vi "SQL读取.vi"(8 "error in (no error)":errorcluster caption="错误输入（无错误）", 10 "ADODB._Connection In":refnum<k7>, 11 "电脑一新返工1":string) -> (0 "error out":errorcluster caption="错误输出", 1 "computer3":string, 2 "computer2":string, 3 "computer1":string, 4 "传递信息显示":string, 5 "ADODB._Connection Out":refnum<k7>)   [LabVIEW 2017]
uses:
  <vilib>/Utility/file.llb/Write Delimited Spreadsheet (string).vi
panel:
  out "工单号":string
  out "元素 3":string
  out "元素 2":string
  out "元素":string
  out "连接的字符串":string
  out "Data":string[][](array[string])
  out "子数组":string[](array[string])
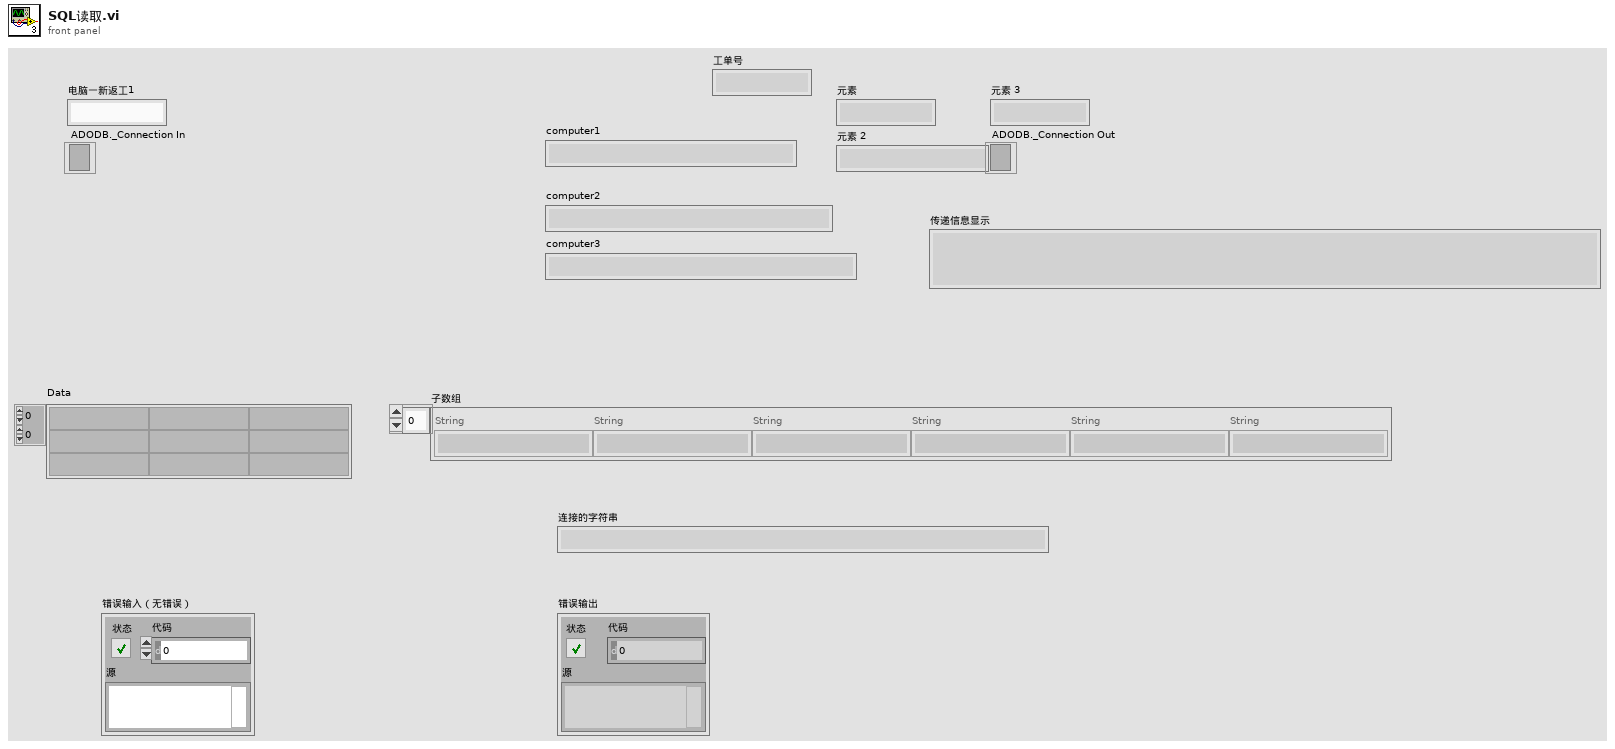
[diagram p1: front panel]
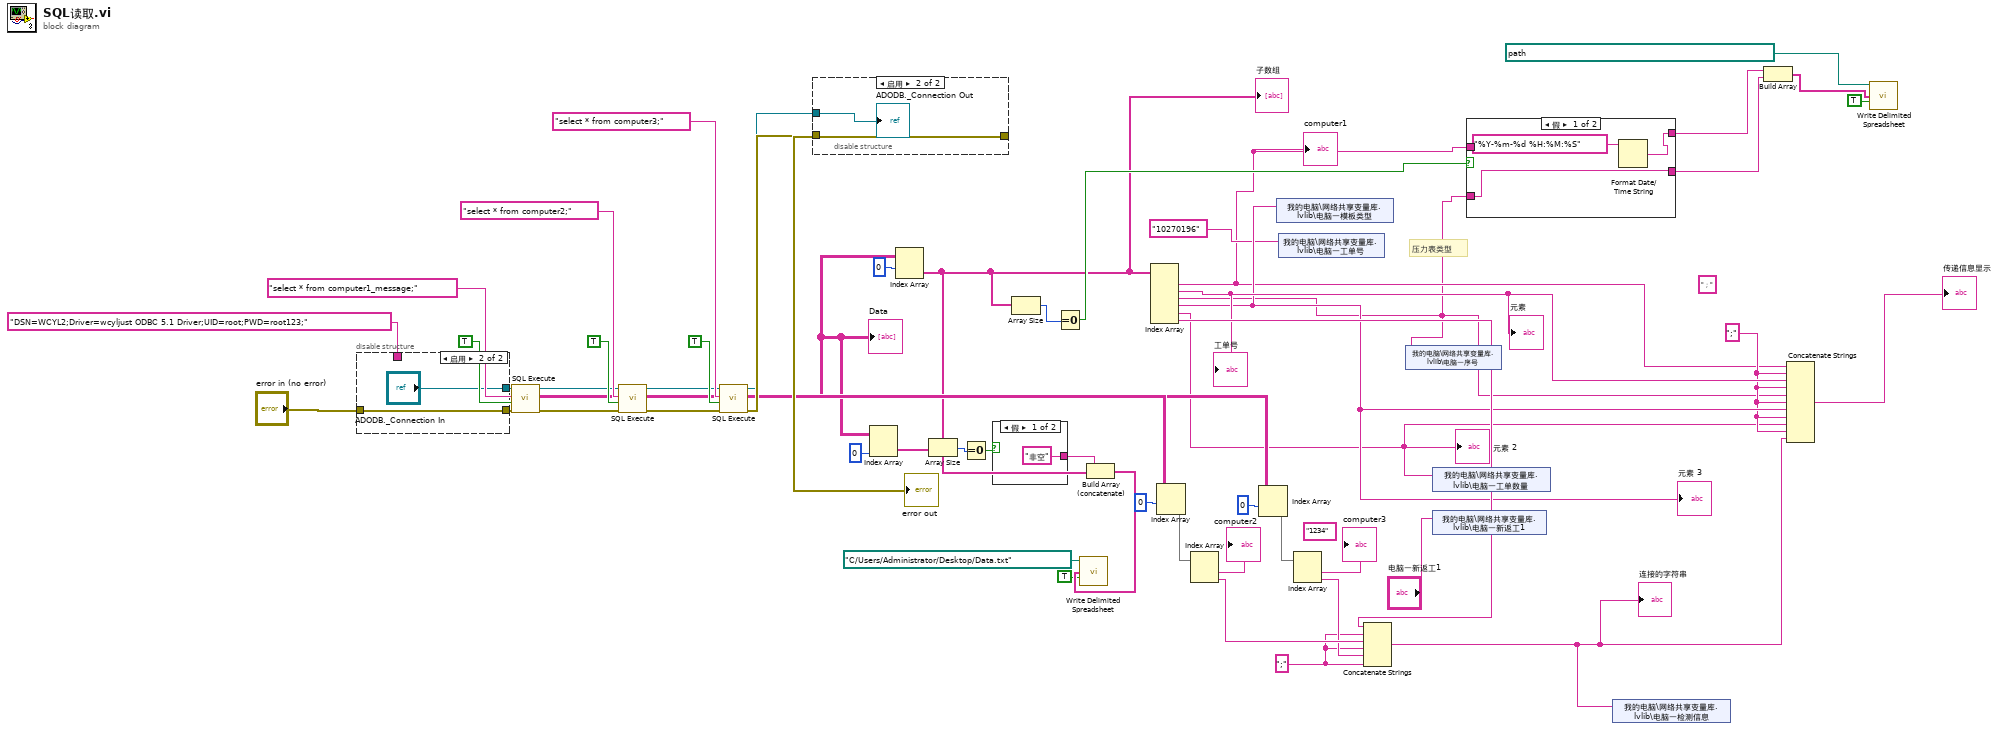
[diagram p0: block diagram]
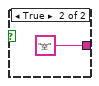
[diagram p2: hidden frame]
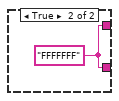
[diagram p3: hidden frame]
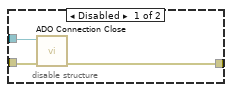
[diagram p4: hidden frame]
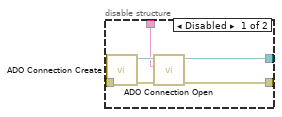
[diagram p5: hidden frame]
diagram:
  (unwired) "1234" ("电脑一返工")
  w22 = ";" ("字符串")
  (unwired) "；" ("字符串")
  w32 = ";" ("字符串")
  # "压力表类型"
  n1 = disable-structure shown="启用" {
    disable-tunnel: "DSN=WCYL2;Driver=wcyljust ODBC 5.1 Driver;UID=root;PWD=root123;" ("ConnectionString") -> [w61 _]
    disable-tunnel: [w60 "ADODB._Connection In"] -> w53
    disable-tunnel: [w59 w65] -> w52
    disable-tunnel: "error in (no error)" -> [w58 w65]
    frame Disabled {
      n2 = call <userlib>:"ADO Connection Create.vi"("error in (no error)"=w58) -> ("error out"=w62:errorcluster, "ADODB._Connection Out"=w63:refnum<k7>)  [unwired: 9 in]
      n3 = call <userlib>:"ADO Connection Open.vi"("error in (no error)"=w62, "ConnectionString"=w61, "ADODB._Connection In"=w63) -> ("error out"=w59:errorcluster, "ADODB._Connection Out"=w60:refnum<k7>)  [unwired: 7 in]
    }
    frame Enabled {
    }
  }
  n4 = call <userlib>:"SQL Execute.vi"("error in (no error)"=w52, "Return Data (T)"=TRUE, "Command Text"="select * from computer1_message;", "ADODB._Connection In"=w53) -> ("error out"=w45:errorcluster, "Data"=w9:string[][], "ADODB._Connection Out"=w42:refnum<k7>)  [unwired: 4 in, 1 out]
  "Data" <- w9
  n5 = call <userlib>:"SQL Execute.vi"("error in (no error)"=w45, "Return Data (T)"=TRUE, "Command Text"="select * from computer2;", "ADODB._Connection In"=w42) -> ("error out"=w44:errorcluster, "Data"=w39:string[][], "ADODB._Connection Out"=w41:refnum<k7>)  [unwired: 4 in, 1 out]
  n6 = call <userlib>:"SQL Execute.vi"("error in (no error)"=w44, "Return Data (T)"=TRUE, "Command Text"="select * from computer3;", "ADODB._Connection In"=w41) -> ("error out"=w43:errorcluster, "Data"=w38:string[][], "ADODB._Connection Out"=w40:refnum<k7>)  [unwired: 4 in, 1 out]
  n7 = disable-structure shown="启用" {
    disable-tunnel: [w68 w70] -> w50
    disable-tunnel: w43 -> [w67 w70]
    disable-tunnel: w40 -> [w66 w69]
    frame Disabled {
      n8 = call <userlib>:"ADO Connection Close.vi"("error in (no error)"=w67, "ADODB._Connection In"=w66) -> ("error out"=w68:errorcluster)  [unwired: 8 in, 1 out]
    }
    frame Enabled {
      "ADODB._Connection Out" <- w69
    }
  }
  "error out" <- w50
  n9 = Index Array(array=w9, index (col)=0 ("禁用的索引 (列)")) -> (element=w7:string[])  [unwired: 1 in]
  n10 = Index Array(array=w9, index (row)=0 ("索引 (行)")) -> (element=w3:string[])  [unwired: 1 in]
  "子数组" <- w3
  n11 = Array Size(array=w7) -> (size(s)=w6:i32)
  n12 = Equal To 0?(x=w6) -> (x = 0?=w5:bool)
  n13 = case shown="假" w5 {
    tunnel: ["非空" "空"] -> w4
    frame False {
    }
    frame True {
    }
  }
  n14 = Array Size(array=w3) -> (size(s)=w16:i32)
  n15 = Equal To 0?(x=w16) -> (x = 0?=w15:bool)
  n16 = Build Array (concatenate)(w4, w3) -> (w2:string[])
  n17 = call-poly <vilib>:"Write Delimited Spreadsheet.vi"("file path (dialog if empty)"=path "C:/Users/Administrator/Desktop/Data.txt", "1D data"=w2, "append to file? (new file:F)"=TRUE) -> ()  [unwired: 11 in, 2 out]
  n18 = Index Array(array=w3) -> (element #1=w14:string, element #2=w36:string, element #3=w12:string, element #4=w33:string, element #5=w31:string, element #6=w37:string)  [unwired: 6 in]
  "computer1" <- w14
  "元素" <- w36
  "元素 2" <- w31
  "元素 3" <- w33
  "工单号" <- w36
  n19 = Index Array(array=w39, index (row)=0 ("索引 (行)")) -> (element=w28:string[])  [unwired: 1 in]
  n20 = Index Array(array=w28) -> (element #1=→"computer2":string, element #2=w26:string)  [unwired: 2 in]
  n21 = Index Array(array=w38, index (row)=0 ("索引 (行)")) -> (element=w27:string[])  [unwired: 1 in]
  n22 = shared-variable "我的电脑\\网络共享变量库.lvlib\\电脑一模板类型"(w33) -> ()  [unwired: 1 in, 1 out]
  n23 = shared-variable "我的电脑\\网络共享变量库.lvlib\\电脑一工单号"("10270196" ("电脑一工单号")) -> ()  [unwired: 1 in, 1 out]
  n24 = Index Array(array=w27) -> (element #1=→"computer3":string, element #2=w25:string)  [unwired: 2 in]
  n25 = Concatenate Strings(w37, w22, w26, w22, w25, w22) -> (w35:string)
  "连接的字符串" <- w35
  n26 = shared-variable "我的电脑\\网络共享变量库.lvlib\\电脑一序号"(w12) -> ()  [unwired: 1 in, 1 out]
  n27 = shared-variable "我的电脑\\网络共享变量库.lvlib\\电脑一工单数量"(w31) -> ()  [unwired: 1 in, 1 out]
  n28 = shared-variable "我的电脑\\网络共享变量库.lvlib\\电脑一新返工1"("电脑一新返工1") -> ()  [unwired: 1 in, 1 out]
  n29 = case shown="假" w15 {
    tunnel: [w73 w76] -> w13
    tunnel: w14 -> [_ _]
    tunnel: [w75 w76] -> w11
    tunnel: w12 -> [w75 _]
    frame False {
      n30 = Format Date/Time String(time format string (%c)="%Y-%m-%d %H:%M:%S" ("时间格式字符串(%c)")) -> (date/time string=w73:string)  [unwired: 2 in]
    }
    frame True {
      w76 = "FFFFFFF" ("String")
    }
  }
  n31 = shared-variable "我的电脑\\网络共享变量库.lvlib\\电脑一检测信息"(w35) -> ()  [unwired: 1 in, 1 out]
  n32 = Build Array(w13, w11) -> (w17:string[])
  n33 = Concatenate Strings(w14, w32, w36, w32, w12, w32, w33, w32, w31, w32, w35) -> (→"传递信息显示":string)
  n34 = call-poly <vilib>:"Write Delimited Spreadsheet.vi"("file path (dialog if empty)"=path "C:/Users/Administrator/Desktop/传递条码信息.txt", "1D data"=w17, "append to file? (new file:F)"=TRUE) -> ()  [unwired: 11 in, 2 out]
